vi "Write Allow Undefined Strings.vi"(8 "error in (no error)":errorcluster, 10 "AllowUndefStrs":bool, 11 "ComboBox.lvclass in":refnum<class "ComboBox.lvclass">) -> (0 "error out":errorcluster, 3 "ComboBox.lvclass out":refnum<class "ComboBox.lvclass">)   [LabVIEW 2015, in "ComboBox.lvclass"]
uses:
  ComboBox.lvclass
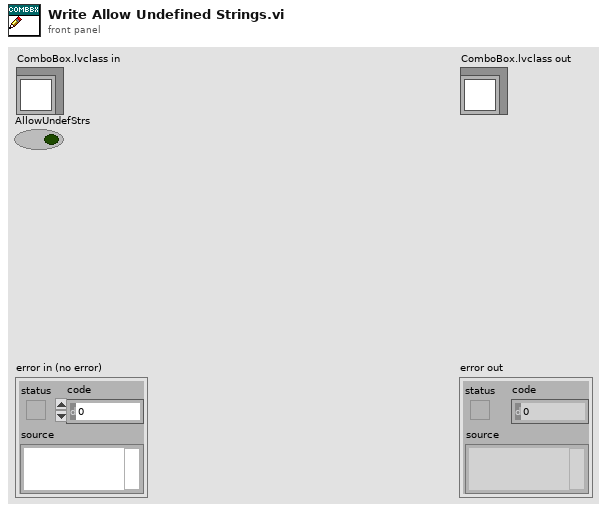
[diagram p1: front panel]
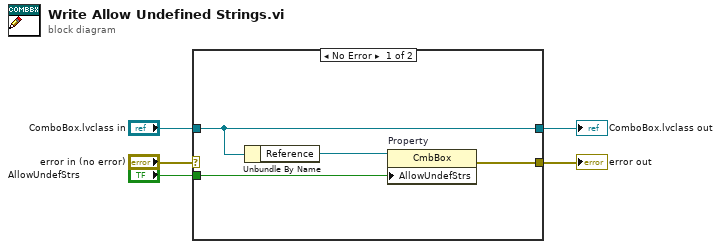
[diagram p0: block diagram]
diagram:
  n1 = case shown="No Error" "error in (no error)" {
    selector: "error in (no error)" -> [_ w11]
    tunnel: [w9 w11] -> w4
    tunnel: [w7 w10] -> w2
    tunnel: "ComboBox.lvclass in" -> [w7 w10]
    tunnel: "AllowUndefStrs" -> [w8 _]
    frame No Error {
      n2 = Unbundle By Name(w7) -> ("Reference"=w6:refnum<vi>)
      n3 = property on="Property" class="CmbBox"(reference=w6, "AllowUndefStrs"=w8) -> (error out=w9:errorcluster)  [unwired: 1 in, 1 out]
    }
    frame Error {
    }
  }
  "error out" <- w4
  "ComboBox.lvclass out" <- w2
